vi "Write bomb status.vi"(8 "error in (no error)":errorcluster, 10 "bomb status":enum16{"none", "exploded", "unexploded"}(ring), 11 "RoomWithABomb in":refnum<class "RoomWithABomb.lvclass">) -> (0 "error out":errorcluster, 3 "RoomWithABomb out":refnum<class "RoomWithABomb.lvclass">)   [LabVIEW 2016, in "RoomWithABomb.lvclass"]
uses:
  RoomWithABomb.lvclass
  RoomWithABomb.lvclass/RoomWithABomb.ctl
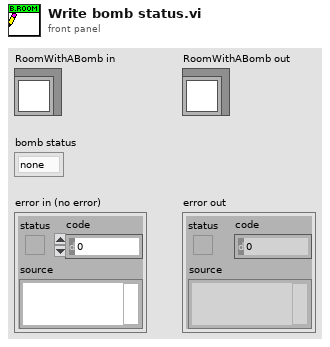
[diagram p1: front panel]
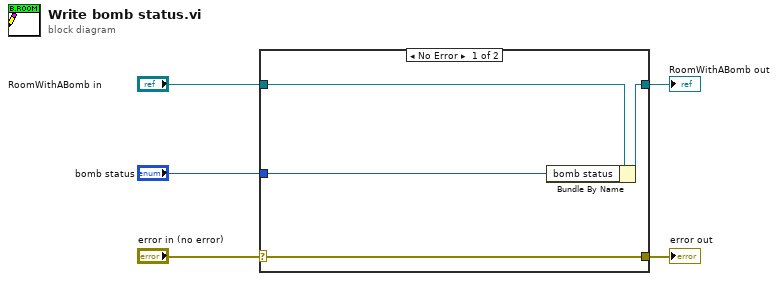
[diagram p0: block diagram]
diagram:
  n1 = case shown="No Error" "error in (no error)" {
    selector: "error in (no error)" -> [w9 w10]
    tunnel: [w9 w10] -> w4
    tunnel: [w7 w11] -> w2
    tunnel: "RoomWithABomb in" -> [w8 w11]
    tunnel: "bomb status" -> [w6 _]
    frame No Error {
      n2 = Bundle By Name(cluster=w8, "bomb status"=w6) -> (w7:refnum<class "RoomWithABomb.lvclass">)
    }
    frame Error {
    }
  }
  "error out" <- w4
  "RoomWithABomb out" <- w2
